vi "Read EventAggregator Enqueuer.vi"(8 "error in (no error)":errorcluster, 11 "IEventHandler in":refnum<class "IEventHandler.lvclass">) -> (0 "error out":errorcluster, 2 "EventAggregator Enqueuer":refnum<class "Message Enqueuer.lvclass">, 3 "IEventHandler out":refnum<class "IEventHandler.lvclass">)   [LabVIEW 2015, in "ActorEvents.lvlib" / "IEventHandler.lvclass"]
uses:
  IEventHandler.lvclass
  <vilib>/ActorFramework/Message Enqueuer/Message Enqueuer.lvclass
  IEventHandler.lvclass/IEventHandler.ctl
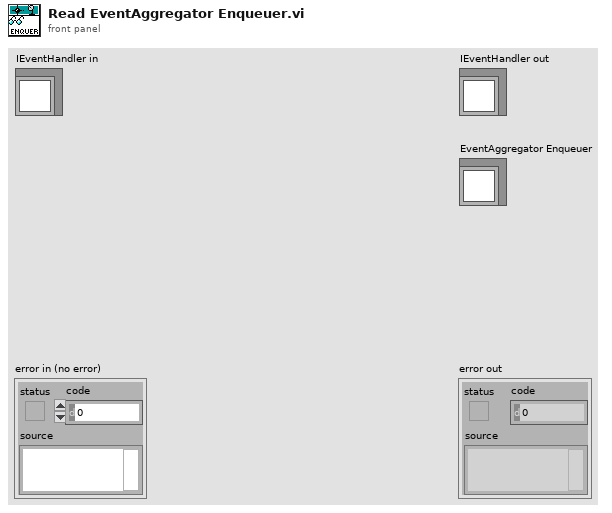
[diagram p1: front panel]
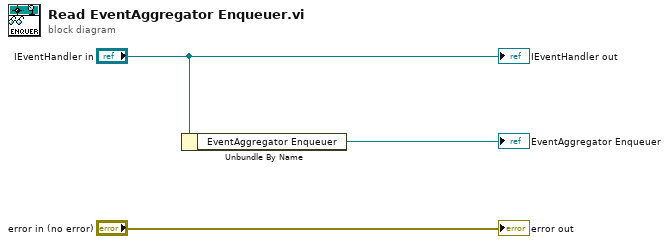
[diagram p0: block diagram]
diagram:
  n1 = Unbundle By Name("IEventHandler in") -> ("EventAggregator Enqueuer"=→"EventAggregator Enqueuer":refnum<class "Message Enqueuer.lvclass">)
  "error out" <- "error in (no error)"
  "IEventHandler out" <- "IEventHandler in"
